vi "MCL Min Max Theta X.vi"(9 "handle":i32, 10 "max":dbl, 11 "min":dbl) -> (1 "function return":i32, 2 "max out":dbl, 3 "min out":dbl)   [LabVIEW 2017, in "Madlib.lvlib"]
doc: "MADLIB_API int MCL_MinMaxThetaX(double *min, double *max, int handle);"
uses:
  Madlib.lvlib
  Madlib.dll
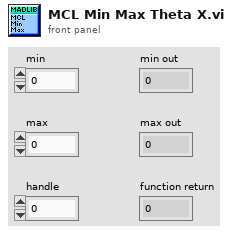
[diagram p1: front panel]
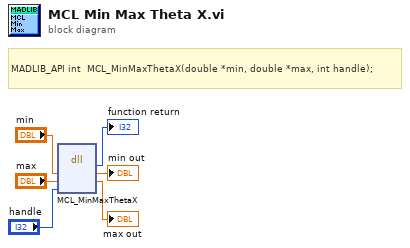
[diagram p0: block diagram]
diagram:
  # "MADLIB_API\tint\t\tMCL_MinMaxThetaX(double *min, double *max, int handle);"
  n1 = dll-call lib="C:/Users/francesco/dev/pump-probe/Piezo/lvlib/Madlib.*" fn="MCL_MinMaxThetaX"("min"="min", "max"="max", "handle"="handle") -> (→"function return":i32, "min"=→"min out":dbl, "max"=→"max out":dbl)  [unwired: 4 in, 2 out]
